vi "Update Parameters Configuration File Error.vi"(8 "error in":errorcluster, 11 "Configuration files Ref":T1 format="%.0x") -> (0 "error out":errorcluster, 3 "Configuration files Ref out":T1 format="%.0x")   [LabVIEW 2020, in "AIM ARINC 429 Scripting.lvlib"]
uses:
  AIM ARINC 429 Scripting.lvlib
  <vilib>/NI VeriStand/Custom Device API/Custom Device Item Ref.ctl
  Constants.vi
  <vilib>/NI VeriStand/Custom Device API/Get Item Property (Boolean).vi
  <vilib>/NI VeriStand/Custom Device API/Custom Device API.lvlib
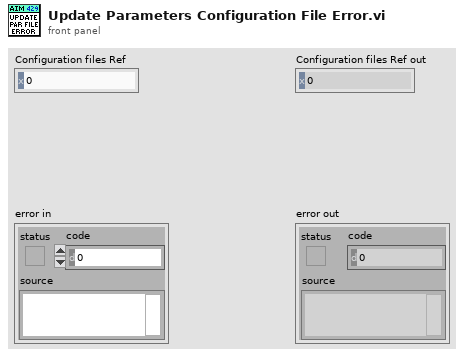
[diagram p1: front panel]
types:
  T1 = typedef "Custom Device API.lvlib/Custom Device Item Ref.ctl" = u64
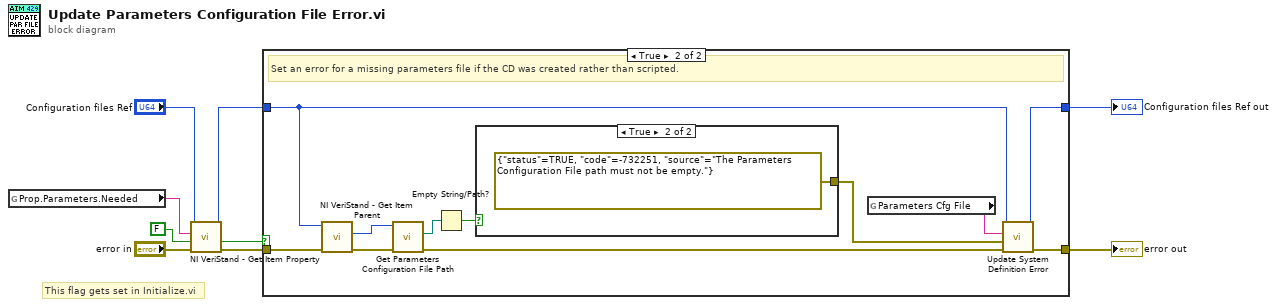
[diagram p0: block diagram]
diagram:
  # "This flag gets set in Initialize.vi"
  n1 = global read "Constants.vi" "Prop.Parameters.Needed"() -> (w1:string)
  n2 = call-poly <vilib>:"NI VeriStand - Get Item Property.vi"("error in (no error)"="error in", "Default Value"=FALSE, "Property Name"=w1, "Item Ref in"="Configuration files Ref") -> ("error out"=w5:errorcluster, "Value"=w7:bool, "Item Ref out"=w3:T1)  [unwired: 4 in, 1 out]
  n3 = case shown="True" w7 {
    tunnel: [w10 w22] -> w9
    tunnel: [w11 w21] -> w8
    tunnel: w5 -> [w11 w13]
    tunnel: w3 -> [w10 w15]
    frame False {
      # "Parameters configuration file is not needed if the CD was scripted."
    }
    frame True {
      # "Set an error for a missing parameters file if the CD was created rather than scripted."
      n4 = call <vilib>:"NI VeriStand - Get Item Parent.vi"("error in (no error)"=w13, "Item Ref in"=w15) -> ("error out"=w14:errorcluster, "Parent Ref"=w16:T1)  [unwired: 6 in, 2 out]
      n5 = call "Get Parameters Configuration File Path.vi"("error in"=w14, "Ballard ARINC 429 custom device in"=w16) -> ("error out"=w19:errorcluster, "parameters configuration file path"=w17:path)  [unwired: 6 in, 2 out]
      n6 = Empty String/Path?(string/path=w17) -> (empty?=w20:bool)
      n7 = case shown="True" w20 {
        tunnel: [_ errorcluster {"status"=TRUE, "code"=-732251, "source"="The Parameters Configuration File path must not be empty."} ("New Error")] -> w18
        frame False {
        }
        frame True {
        }
      }
      n8 = global read "Constants.vi" "Parameters Cfg File"() -> (w12:string)
      n9 = call "Update System Definition Error.vi"("error to report"=w19, "error in"=w18, "error key"=w12, "Configuration files Ref"=w15) -> ("error out"=w21:errorcluster, "Configuration files Ref out"=w22:T1)  [unwired: 6 in]
    }
  }
  "error out" <- w8
  "Configuration files Ref out" <- w9
